vi "Get Rotate Temp(SubVI).vi"(11 ".NET引用句柄输入":refnum<k24>) -> (3 "Result":dbl)   [LabVIEW 2019, in "User lib.lvlib"]
uses:
  User lib.lvlib
  lib/QDInstrument.dll
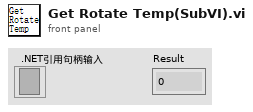
[diagram p1: front panel]
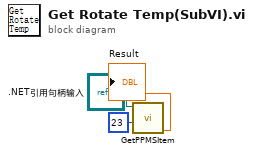
[diagram p0: block diagram]
diagram:
  n1 = call "GetPPMSItem.vi"("Channel"=23, "Instrument Ref In"=".NET引用句柄输入") -> ("Result"=→"Result":dbl)  [unwired: 2 in, 3 out]
